vi "flicker test with zero - explicit scope settings.vi"() -> ()   [LabVIEW 2011]
uses:
  <instrlib>/Tektronix DPO MSO 2000 4000 Series/Public/Configure/Configure Trigger (Edge).vi
  <instrlib>/Tektronix DPO MSO 2000 4000 Series/Public/Data/Read (Single Waveform).vi
  <instrlib>/Tektronix DPO MSO 2000 4000 Series/Tektronix DPO MSO 2000 4000 Series.lvlib
panel:
  in  "Amp gain":string
  in  "Test repeat #":string
  in  "Dim level% (eg. \"025\"))":string
  in  "Dimmer type (eg. \"x\")":string
  in  "Model (eg. \"omni05\")":string
  in  "Channel (0: Channel 1)":u16(ring) items=["Channel 1", "Channel 2", "Channel 3", "Channel 4", "Math", "Reference 1", "Reference 2", "Reference 3", "Reference 4", "D0", "D1", "D2", "D3", "D4", "D5", "D6", "D7", "D8", "D9", "D10", "D11", "D12", "D13", "D14", "D15", "Amplitude", "Frequency", "Phase", "Normal", "Average", "Maximum Peak Hold", "Minimum Peak Hold"]
  in  "Maximum Time (10000ms)":u32=10000
  in  "VISA Resource Name":refnum<visa-resource-name>
  out "Filename Out":path
  out "appended path":path
  out "data":waveform(dbl)(graph)
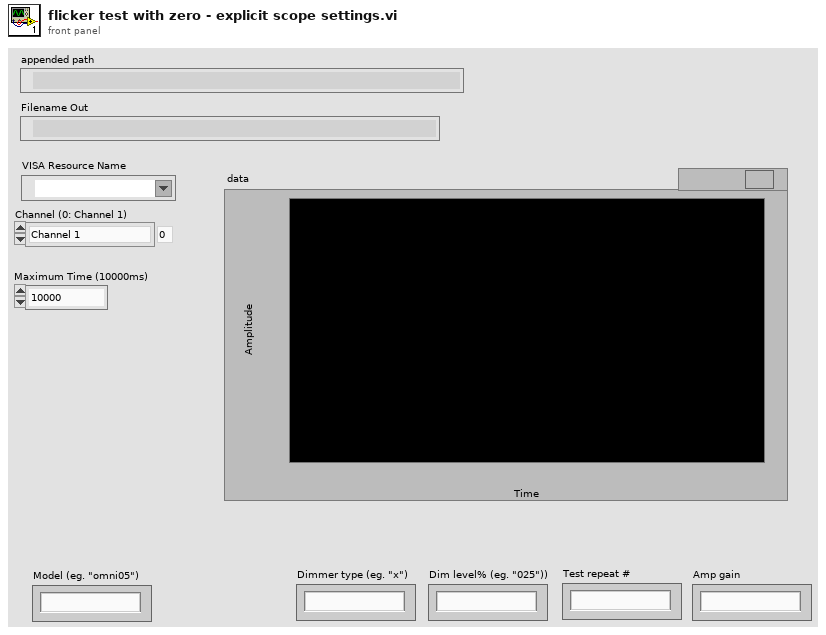
[diagram p1: front panel]
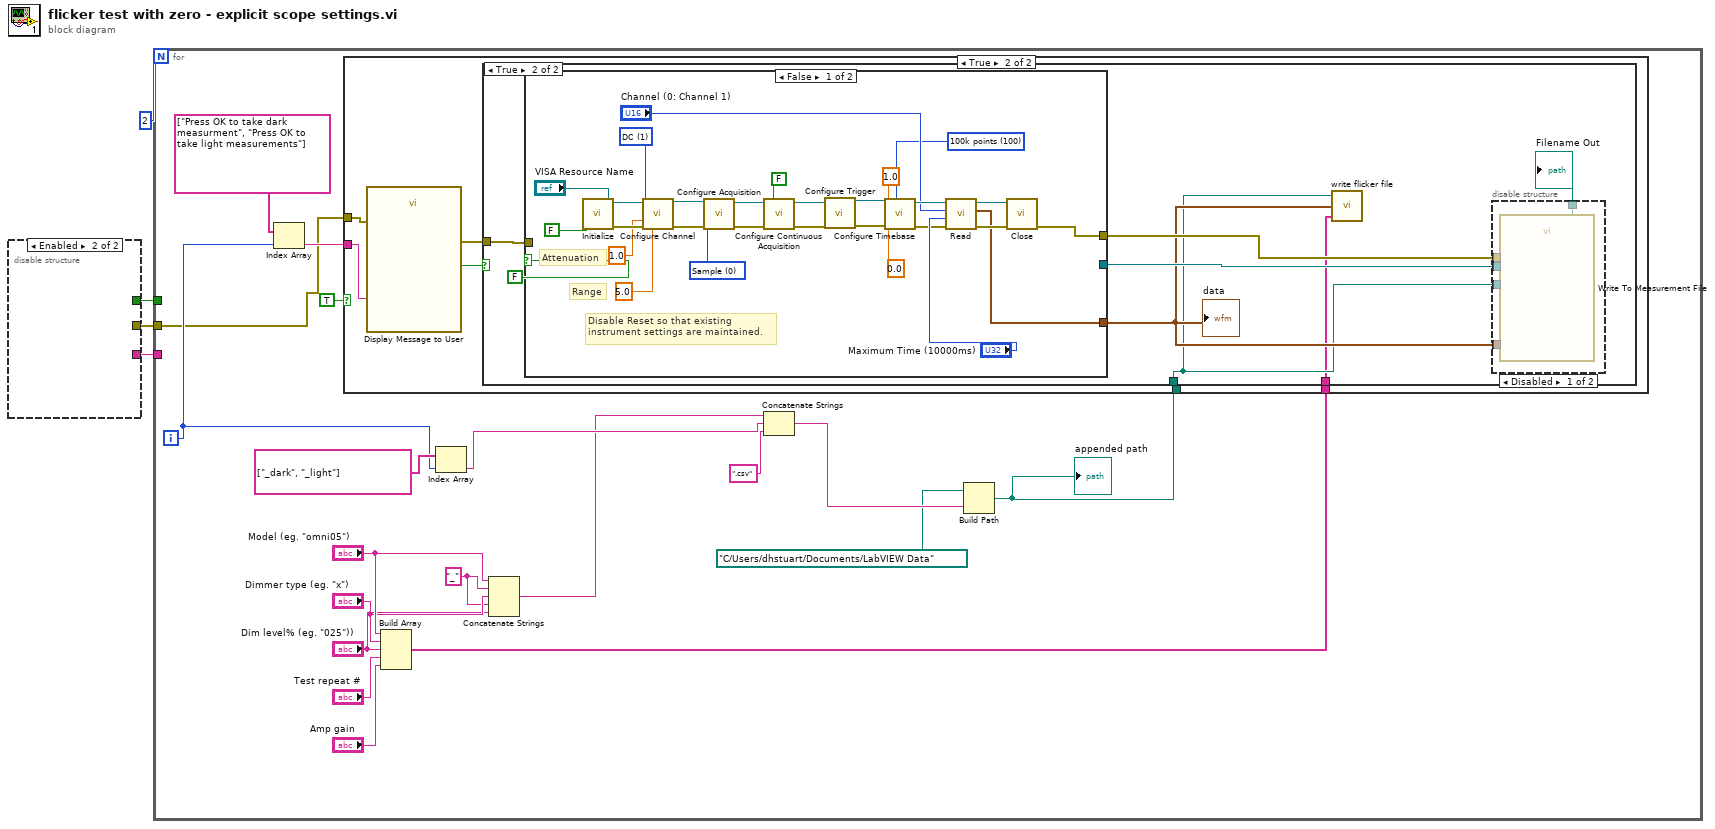
[diagram p0: block diagram]
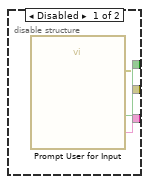
[diagram p2: hidden frame]
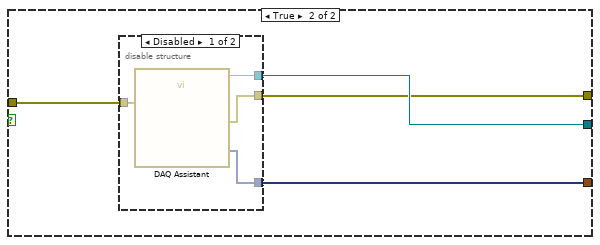
[diagram p6: hidden frame]
diagram:
  n1 = disable-structure shown="Enabled" {
    disable-tunnel: [w7 _] -> w3
    disable-tunnel: [w6 _] -> w2
    disable-tunnel: [w5 _] -> w1
    frame Disabled {
      n2 = call "Prompt User for Input"() -> ("file_name"=w7:string, "OK"=w6:bool, "error out"=w5:errorcluster)  [unwired: 17 in]
    }
    frame Enabled {
    }
  }
  n3 = for {
    N: 2 -> [_]
    tunnel: w3 -> [_]
    tunnel: w2 -> [_]
    tunnel: w1 -> [w17]
    i -> [w21]
    w12 = "_"
    n4 = Index Array(array=string[] ["Press OK to take dark measurment", "Press OK to take light measurements"], index=w21) -> (element=w25:string)
    n5 = Build Array("Model (eg. \"omni05\")", "Dimmer type (eg. \"x\")", "Dim level% (eg. \"025\"))", "Test repeat #", "Amp gain") -> (w8:string[])
    n6 = Index Array(array=string[] ["_dark", "_light"], index=w21) -> (element=w19:string)
    n7 = Concatenate Strings("Model (eg. \"omni05\")", w12, "Dimmer type (eg. \"x\")", w12, "Dim level% (eg. \"025\"))") -> (w10:string)
    n8 = Concatenate Strings(w10, w19, ".csv" ("string")) -> (w24:string)
    n9 = Build Path(base path=path "C:/Users/dhstuart/Documents/LabVIEW Data", name or relative path=w24) -> (appended path=w23:path)
    "appended path" <- w23
    n10 = case shown="True" TRUE {
      tunnel: w25 -> [_ w30]
      tunnel: w23 -> [_ w29]
      tunnel: w17 -> [_ w28]
      tunnel: w8 -> [_ w27]
      frame False {
      }
      frame True {
        n11 = call "Display Message to User"("error in (no error)"=w28, "Message"=w30) -> ("error out"=w32:errorcluster, "OK"=w31:bool)  [unwired: 8 in]
        n12 = case shown="True" w31 {
          tunnel: w32 -> [_ w40]
          tunnel: w29 -> [_ w34]
          tunnel: w27 -> [_ w33]
          frame False {
          }
          frame True {
            n13 = case shown="False" FALSE {
              tunnel: w40 -> [_ w77]
              tunnel: [_ w76] -> w39
              tunnel: [w68 w75] -> w35
              tunnel: [w67 w74] -> w38
              frame False {
                w48 = u16 1 items=["AC", "DC", "Ground"] ("Vertical Coupling (1: DC)")
                w49 = u32 100 items=["1000 points"=1, "10k points"=10, "100k points"=100, "1M points"=1000, "5M points"=5000, "10M points"=10000] ("Record Length (10: 10k points)")
                w54 = u16 0 items=["Sample", "Peak Detect", "Hi Res", "Envelope", "Average"] ("Acquisition Type (0: Sample)")
                # "Range"
                # "Attenuation"
                # "Disable Reset so that existing\ninstrument settings are maintained."
                n14 = call <instrlib>:"Initialize.vi"("Reset (True)"=FALSE ("Reset? (T: Yes)"), "VISA resource name"="VISA Resource Name") -> ("error out"=w60:errorcluster, "VISA resource name out"=w66:refnum<visa-resource-name>)  [unwired: 8 in]
                n15 = call <instrlib>:"Configure Channel.vi"("VISA resource name"=w66, "Vertical Coupling (1: DC)"=w48, "Probe Attenuation (1)"=1.0, "error in (no error)"=w60, "Vertical Range (10.0 V)"=5.0) -> ("VISA resource name out"=w65:refnum<visa-resource-name>, "error out"=w59:errorcluster)  [unwired: 9 in]
                n16 = call <instrlib>:"Configure Acquisition.vi"("error in (no error)"=w59, "Acquisition Type (0: Sample)"=w54, "VISA resource name"=w65) -> ("error out"=w58:errorcluster, "VISA resource name out"=w64:refnum<visa-resource-name>)  [unwired: 7 in]
                n17 = call <instrlib>:"Configure Continuous Acquisition.vi"("error in (no error)"=w58, "Enable Continuous Acquisition Mode (T: Enable)"=FALSE, "VISA resource name"=w64) -> ("error out"=w57:errorcluster, "VISA resource name out"=w63:refnum<visa-resource-name>)  [unwired: 7 in]
                n18 = call-poly <instrlib>:"Configure Trigger.vi"("VISA resource name"=w63, "error in (no error)"=w57) -> ("VISA resource name out"=w62:refnum<visa-resource-name>, "error out"=w56:errorcluster)  [unwired: 12 in]
                n19 = call <instrlib>:"Configure Timebase.vi"("Record Length (10: 10k points)"=w49, "error in (no error)"=w56, "Position (10 %)"=0.0, "Timebase (0.0005 s)"=1.0, "VISA resource name"=w62) -> ("error out"=w55:errorcluster, "VISA resource name out"=w61:refnum<visa-resource-name>)  [unwired: 5 in]
                n20 = call-poly <instrlib>:"Read.vi"("error in (no error)"=w55, "Maximum Time (10000ms)"="Maximum Time (10000ms)", "Channel (0: Channel 1)"="Channel (0: Channel 1)", "VISA resource name"=w61) -> ("error out"=w71:errorcluster, "Waveform Graph"=w68:waveform(dbl), "VISA resource name out"=w69:refnum<visa-resource-name>)  [unwired: 5 in]
                n21 = call <instrlib>:"Close.vi"("error in (no error)"=w71, "VISA resource name"=w69) -> ("error out"=w67:errorcluster)  [unwired: 9 in]
              }
              frame True {
                n22 = disable-structure shown="Disabled" {
                  disable-tunnel: w77 -> [w81 _]
                  disable-tunnel: [w80 _] -> w76
                  disable-tunnel: [w79 _] -> w75
                  disable-tunnel: [w78 _] -> w74
                  frame Disabled {
                    n23 = call "DAQ Assistant"("error in"=w81) -> ("task out"=w80:refnum<k21>, "data"=w79:dynamicdata, "error out"=w78:errorcluster)  [unwired: 16 in]
                  }
                  frame Enabled {
                  }
                }
              }
            }
            "data" <- w35
            n24 = call "write flicker file.vi"("Array"=w33, "Waveform Data"=w35, "appended path"=w34) -> ()  [unwired: 1 in]
            n25 = disable-structure shown="Disabled" {
              disable-tunnel: w39 -> [w45 _]
              disable-tunnel: w35 -> [w44 _]
              disable-tunnel: w38 -> [w43 _]
              disable-tunnel: w34 -> [w42 _]
              disable-tunnel: [w41 _] -> w37
              frame Disabled {
                n26 = call "Write To Measurement File"("Signals"=w44, "error in (no error)"=w43, "Filename"=w42, "DAQmx Task"=w45) -> ("Filename Out"=w41:path)  [unwired: 13 in, 2 out]
              }
              frame Enabled {
              }
            }
            "Filename Out" <- w37
          }
        }
      }
    }
  }
